vi "SanityCheck.vi"(8 "error in (no error)":errorcluster, 11 "CDependencyList in":refnum<class "CDependencyList.lvclass">) -> (0 "error out":errorcluster, 1 "Failed checks":string, 3 "CDependencyList out":refnum<class "CDependencyList.lvclass">)   [LabVIEW 2020, in "DependencyInspection.lvlib" / "CDependencyList.lvclass"]
uses:
  CDependencyList/CDependencyList.lvclass
  obj/Addons/LabVIEWObjectInterfaces.lvlibp/LabVIEWObjectInterfaces/ILabVIEWItem/ILabVIEWItem.lvclass
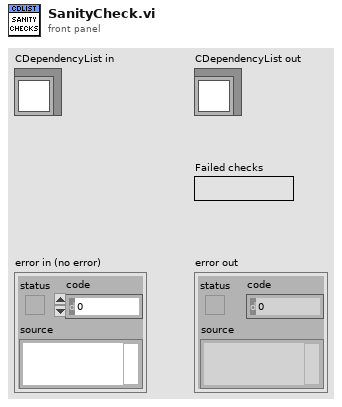
[diagram p1: front panel]
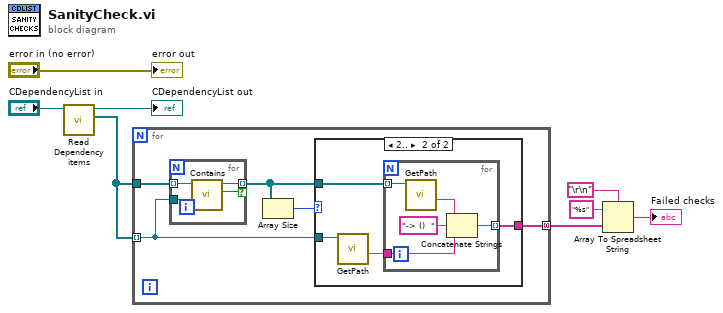
[diagram p0: block diagram]
diagram:
  n1 = call-dynamic "Read Dependency items.vi"("CDependencyList in"="CDependencyList in") -> ("Dependency items"=w1:refnum<class "ILabVIEWItem.lvclass">[], "CDependencyList out"=→"CDependencyList out":refnum<class "CDependencyList.lvclass">)  [unwired: 9 in]
  n2 = for {
    tunnel: w1 -> [w9] mode=indexing
    tunnel: w1 -> [w13]
    tunnel: [w10] -> w7 mode=concatenating
    n3 = for {
      tunnel: w13 -> [w14] mode=indexing
      tunnel: w9 -> [w17]
      tunnel: [w16] -> w11 mode=indexing if=w15
      n4 = call-dynamic "Contains.vi"("Item"=w17, "ILabVIEWItem in"=w14) -> ("Contains?"=w15:bool, "ILabVIEWItem out"=w16:refnum<class "ILabVIEWItem.lvclass">)  [unwired: 7 in, 1 out]
    }
    n5 = Array Size(array=w11) -> (size(s)=w12:i32)
    n6 = case shown="2.." w12 {
      tunnel: w9 -> [_ w20]
      tunnel: w11 -> [_ w21]
      tunnel: [_ w18] -> w10
      frame Default {
      }
      frame 2.. {
        n7 = call-dynamic "GetPath.vi"("ILabVIEWItem in"=w20) -> ("Path"=w19:string)  [unwired: 8 in, 2 out]
        n8 = for {
          tunnel: w21 -> [w26] mode=indexing
          tunnel: w19 -> [w23]
          tunnel: [w22] -> w18 mode=indexing
          n9 = call-dynamic "GetPath.vi"("ILabVIEWItem in"=w26) -> ("Path"=w25:string)  [unwired: 8 in, 2 out]
          n10 = Concatenate Strings(w25, "-> ()  " ("string"), w23) -> (w22:string)
        }
      }
    }
  }
  n11 = Array To Spreadsheet String(delimiter (Tab)="\r\n", array=w7, 3:"%s" ("format string")) -> (spreadsheet string=→"Failed checks":string)
  "error out" <- "error in (no error)"
